vi "WriteToFile.vi"(0 "object in":refnum<class "ErrorLogFile.lvclass">, 2 "Count":i32, 3 "ReportedError":errorcluster, 5 "Error In":errorcluster) -> (14 "object out":refnum<class "ErrorLogFile.lvclass">, 19 "Error Out":errorcluster)   [LabVIEW 2018, in "ErrorLogFile.lvclass"]
uses:
  ErrorLogFile.lvclass
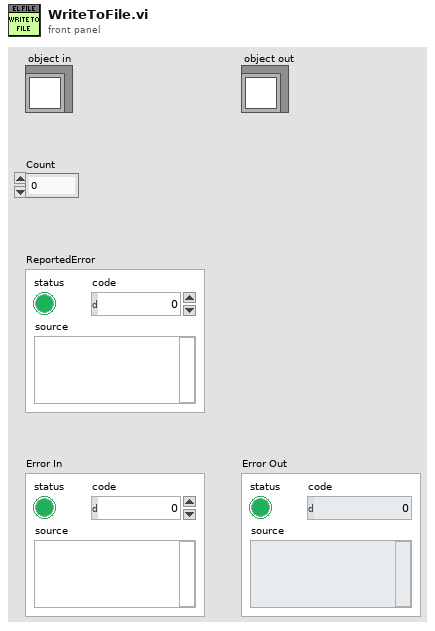
[diagram p1: front panel]
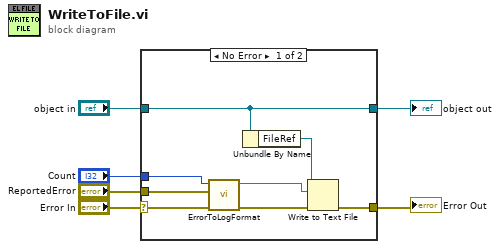
[diagram p0: block diagram]
diagram:
  n1 = case shown="No Error" "Error In" {
    selector: "Error In" -> [w9 w16]
    tunnel: [w12 w16] -> w5
    tunnel: [w14 w15] -> w3
    tunnel: "object in" -> [w14 w15]
    tunnel: "ReportedError" -> [w10 _]
    tunnel: "Count" -> [w13 _]
    frame No Error {
      n2 = call "ErrorToLogFormat.vi"("error in (no error)"=w9, "ReportedError"=w10, "Count"=w13) -> ("error out"=w8:errorcluster, "Log format"=w7:string)  [unwired: 7 in]
      n3 = Unbundle By Name(w14) -> ("FileRef"=w11:refnum<file>)
      n4 = Write to Text File(file (use dialog)=w11, text=w7, error in=w8) -> (error out=w12:errorcluster)  [unwired: 1 in, 2 out]
    }
    frame Error {
    }
  }
  "Error Out" <- w5
  "object out" <- w3
